vi "example_04_decimation_values.vi"() -> ()   [LabVIEW 2015, in "lv-graph.lvlib"]
uses:
  public/_controls/decimation_type.ctl
  public/advanced/build_graph-single_axis.vi
  public/advanced/decimate-value_single_axis.vi
  lv-graph.lvlib
panel:
  in  "outlier_value":dbl=100.0 format="%#_13g"
  in  "outliers":i32=1000
  in  "interval":dbl=10.0 format="%#_13g"
  in  "data_to_generate":i32=100
  out "data_decimated":T1(graph)
  in  "stop":bool
  in  "decimation_type":T2
  in  "decimate_data":bool
  out "data_raw":T1(graph)
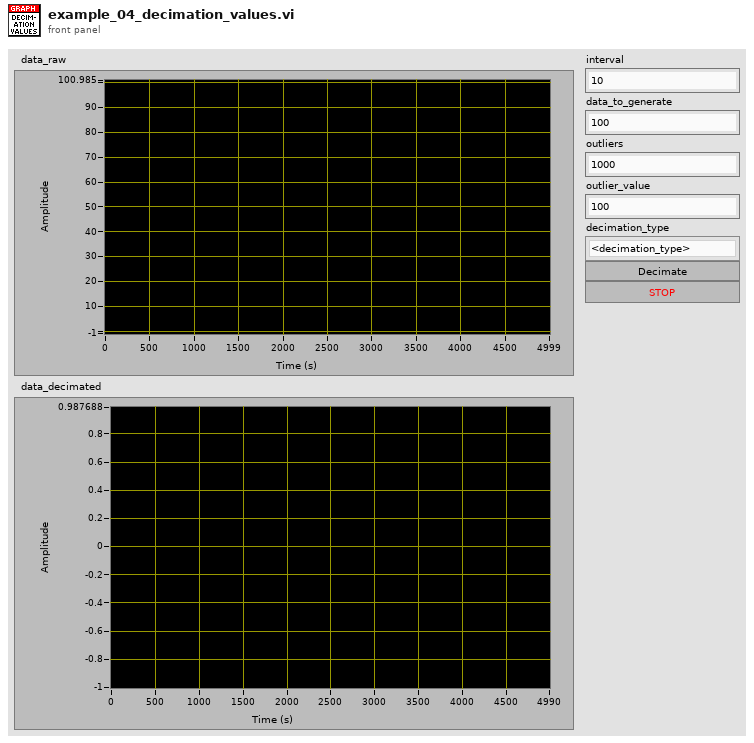
[diagram p1: front panel]
types:
  T1 = cluster{"Time [] out":dbl[], "Data[][] out":dbl[]}[]
  T2 = typedef "lv-graph.lvlib/decimation_type.ctl" = enum16{"<decimation_type>", "average", "min_max", "max", "min", "first", "last"}
  T3 = cluster{"x_scale_maximum":dbl, "x_scale_minimum":dbl, "y_scale_maximum":dbl, "y_scale_minimum":dbl}
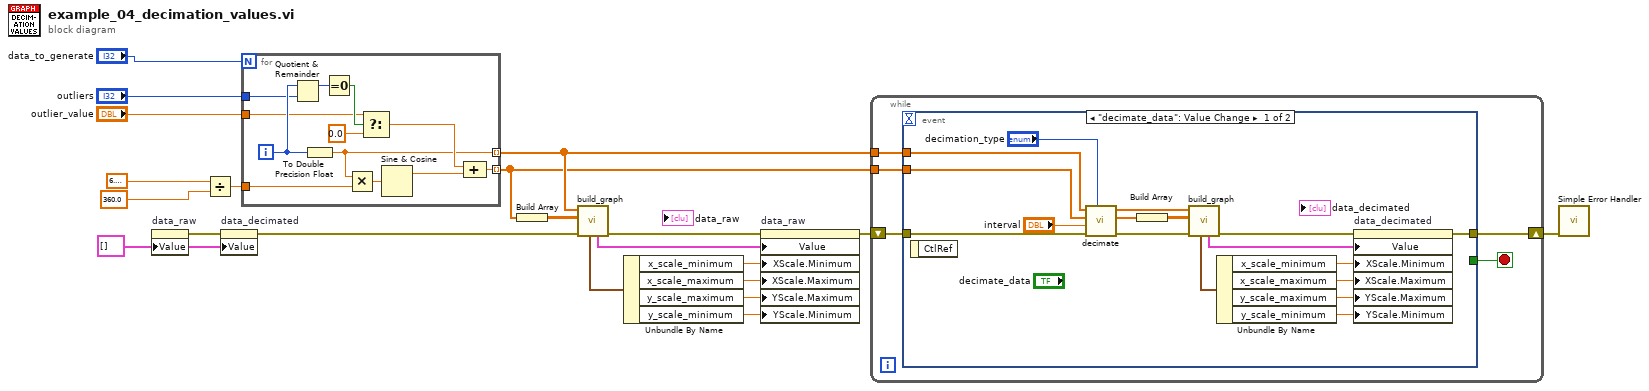
[diagram p0: block diagram]
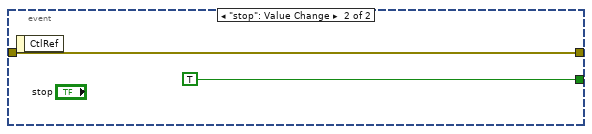
[diagram p2: hidden frame]
diagram:
  w9 = T1 [] ("Graph")
  n1 = property on="data_raw" class="XYGraph (strict)"("Value"=w9) -> (error out=w11:errorcluster)  [unwired: 2 in, 1 out]
  n2 = Divide(x=6.283185307179586, y=360.0) -> (x/y=w20:dbl)
  n3 = property on="data_decimated" class="XYGraph (strict)"(error in=w11, "Value"=w9) -> (error out=w10:errorcluster)  [unwired: 1 in, 1 out]
  n4 = for {
    N: "data_to_generate" -> [_]
    tunnel: w20 -> [w33]
    tunnel: [w28] -> w4 mode=indexing
    tunnel: [w29] -> w8 mode=indexing
    tunnel: "outliers" -> [w23]
    tunnel: "outlier_value" -> [w22]
    i -> [w26]
    n5 = Quotient & Remainder(x=w26, y=w23) -> (x-y*floor(x/y)=w25:i32)  [unwired: 1 out]
    n6 = To Double Precision Float(number=w26) -> (double precision float=w29:dbl)
    n7 = Equal To 0?(x=w25) -> (x = 0?=w24:bool)
    n8 = Multiply(x=w29, y=w33) -> (x*y=w32:dbl)
    n9 = Select(t=w22, s=w24, f=0.0) -> (s? t:f=w30:dbl)
    n10 = Sine & Cosine(0:w32) -> (1:w31:dbl)  [unwired: 1 out]
    n11 = Compound Arithmetic op=ADD(w30, w31) -> (w28:dbl)
  }
  n12 = Build Array(w4) -> (w7:dbl[][])
  n13 = call-poly "build_graph.vi"("error in (no error)"=w10, "y_axis"=w7, "x_axis"=w8) -> ("error out"=w15:errorcluster, "graph_data"=w5:cluster{dbl[], dbl[]}[], "scale_ranges"=w6:T3)  [unwired: 6 in]
  n14 = Unbundle By Name(w6) -> ("x_scale_minimum"=w17:dbl, "x_scale_maximum"=w16:dbl, "y_scale_maximum"=w18:dbl, "y_scale_minimum"=w19:dbl)
  n15 = property on="data_raw" class="XYGraph (strict)"(error in=w15, "Value"=w5, "XScale.Minimum"=w17, "XScale.Maximum"=w16, "YScale.Maximum"=w18, "YScale.Minimum"=w19) -> (error out=w14:errorcluster)  [unwired: 1 in, 1 out]
  n16 = while {
    shift-right: [w36] -> w13
    shift-left: w14 -> [w38]
    tunnel: w8 -> [w35]
    tunnel: w4 -> [w34]
    stop <- w37 stop-if-true
    n17 = event shown="[0] \"decimate_data\": Value Change" {
      selector: _ -> [_ _]
      dyn-events: _ -> [_ _]
      timeout: _ -> [_ _]
      tunnel: w38 -> [w54 w56]
      tunnel: [_ TRUE] -> w37
      tunnel: [w47 w56] -> w36
      tunnel: w35 -> [w40 _]
      tunnel: w34 -> [w41 _]
      event "decimate_data": Value Change {
        n18 = event-data() -> ()  [unwired: 1 in, 1 out]
        n19 = call-poly "decimate.vi"("type"="decimation_type", "error in (no error)"=w54, "interval"="interval", "y_axis in"=w41, "x_axis in"=w40) -> ("error out"=w53:errorcluster, "y_axis out"=w45:dbl[], "x_axis out"=w46:dbl[])  [unwired: 4 in]
        n20 = Build Array(w45) -> (w42:dbl[][])
        n21 = call-poly "build_graph.vi"("error in (no error)"=w53, "y_axis"=w42, "x_axis"=w46) -> ("error out"=w55:errorcluster, "graph_data"=w43:cluster{dbl[], dbl[]}[], "scale_ranges"=w44:T3)  [unwired: 6 in]
        n22 = Unbundle By Name(w44) -> ("x_scale_minimum"=w50:dbl, "x_scale_maximum"=w49:dbl, "y_scale_maximum"=w51:dbl, "y_scale_minimum"=w52:dbl)
        n23 = property on="data_decimated" class="XYGraph (strict)"(error in=w55, "Value"=w43, "XScale.Minimum"=w50, "XScale.Maximum"=w49, "YScale.Maximum"=w51, "YScale.Minimum"=w52) -> (error out=w47:errorcluster)  [unwired: 1 in, 1 out]
      }
      event "stop": Value Change {
        n24 = event-data() -> ()  [unwired: 1 in, 1 out]
      }
    }
  }
  n25 = call <vilib>:"Simple Error Handler.vi"("error in (no error)"=w13) -> ()  [unwired: 4 in, 5 out]
